vi "Teste_comunicação_PC.vi"() -> ()   [LabVIEW 2017]
panel:
  in  "Estado_esteira":bool
  in  "Stop Button":bool
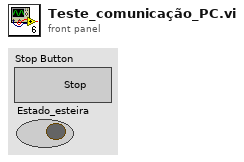
[diagram p1: front panel]
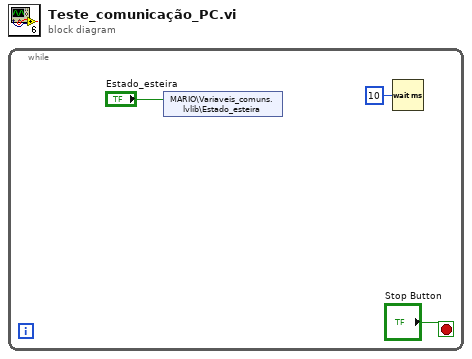
[diagram p0: block diagram]
diagram:
  n1 = while {
    stop <- "Stop Button" stop-if-true
    n2 = shared-variable "MARIO\\Variaveis_comuns.lvlib\\Estado_esteira"("Estado_esteira") -> ()  [unwired: 1 in, 1 out]
    n3 = Wait (ms)(milliseconds to wait=u32 10) -> ()  [unwired: 1 out]
  }
